vi "MusicLoad.vi"(8 "error in (no error)":errorcluster, 11 "path":path) -> (0 "error out":errorcluster)   [LabVIEW 2015, in "LabBASSMOD2.lvlib"]
uses:
  LabBassMOD2.lvlib
  DLL/BASSMOD.dll
panel:
  out "Return":i32
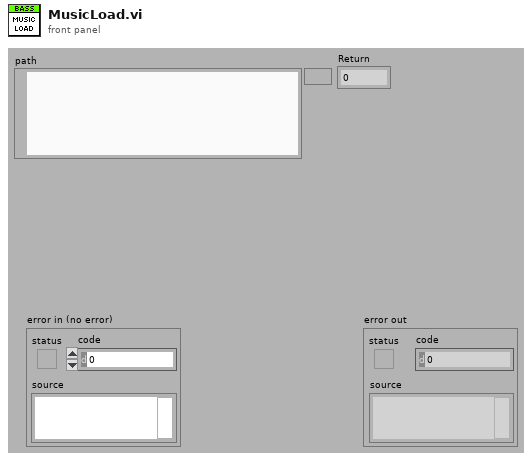
[diagram p1: front panel]
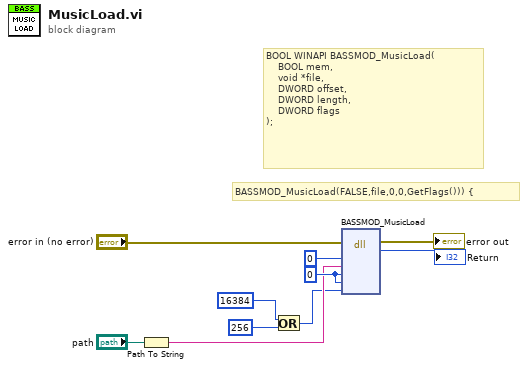
[diagram p0: block diagram]
diagram:
  w9 = u32 0 ("offset")
  # "BOOL WINAPI BASSMOD_MusicLoad(\n    BOOL mem,\n    void *file,\n    DWORD offset,\n    DWORD length,\n    DWORD flags\n);"
  # "BASSMOD_MusicLoad(FALSE,file,0,0,GetFlags())) {"
  n1 = Path To String(path="path") -> (string=w8:string)
  n2 = Or(x=u32 16384 ("flags"), y=u32 256 ("flags")) -> (x .or. y?=w5:u32)
  n3 = dll-call lib="C:/dev/PGS/LabBASSMOD2/DLL/BASSMOD.dll" fn="BASSMOD_MusicLoad"(error in="error in (no error)", "mem"=0, "file"=w8, "offset"=w9, "length"=w9, "flags"=w5) -> (error out=→"error out":errorcluster, "return type"=→"Return":i32)  [unwired: 7 in, 1 out]
